vi "Calc Load.vi"(11 "[A/D]":dbl[](array[numeric])) -> (0 "Loads":dbl[](array[numeric]), 1 "Condyle B Load":dbl, 2 "Condyle A Load":dbl, 3 "Total Load":dbl)   [LabVIEW 2015]
uses:
  <vilib>/gmath/NI_Gmath.lvlib
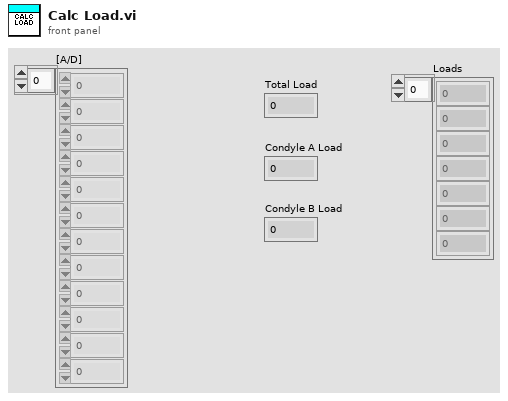
[diagram p1: front panel]
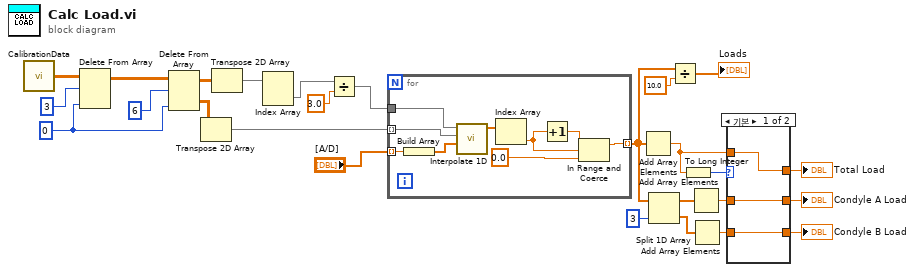
[diagram p0: block diagram]
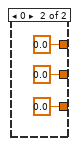
[diagram p2: hidden frame]
diagram:
  w26 = 0 ("index")
  n1 = call "CalibrationData.vi"() -> ("CalData Out"=w4:dbl[][])  [unwired: 1 in]
  n2 = Delete From Array(array=w4, length=3 ("index"), index (col)=w26) -> (array with subset deleted=w24:dbl[][])  [unwired: 1 in, 1 out]
  n3 = Delete From Array(array=w24, length=6, index (col)=w26) -> (deleted portion=w5:dbl[][], array with subset deleted=w22:dbl[][])  [unwired: 1 in]
  n4 = Transpose 2D Array(2D array=w5) -> (transposed array=w18:dbl[][])
  n5 = Transpose 2D Array(2D array=w22) -> (transposed array=w19:dbl[][])
  n6 = Index Array(array=w19) -> (element=w20:dbl[])  [unwired: 2 in]
  n7 = Divide(x=w20, y=3.0 ("Numeric")) -> (x/y=w17:dbl[])
  n8 = for {
    tunnel: w17 -> [w35]
    tunnel: "[A/D]" -> [w34] mode=indexing
    tunnel: [w29] -> w3 mode=indexing
    tunnel: w18 -> [w28] mode=indexing
    n9 = Build Array(w34) -> (w33:dbl[])
    n10 = call <vilib>:"Interpolate 1D.vi"("xi"=w33, "X"=w28, "Y"=w35) -> ("yi"=w32:dbl[])  [unwired: 6 in, 2 out]
    n11 = Index Array(array=w32) -> (element=w31:dbl)  [unwired: 1 in]
    n12 = Increment(x=w31) -> (x+1=w27:dbl)
    n13 = In Range and Coerce(upper limit=w27, x=w31, lower limit=0.0) -> (coerced(x)=w29:dbl)  [unwired: 1 out]
  }
  n14 = Add Array Elements(numeric array=w3) -> (sum=w15:dbl)
  n15 = Split 1D Array(array=w3, index=3) -> (first subarray=w11:dbl[], second subarray=w10:dbl[])
  n16 = Divide(x=w3, y=10.0 ("lower limit")) -> (x/y=→"Loads":dbl[])
  n17 = To Long Integer(number=w15) -> (32bit integer=w16:i32)
  n18 = Add Array Elements(numeric array=w11) -> (sum=w9:dbl)
  n19 = Add Array Elements(numeric array=w10) -> (sum=w8:dbl)
  n20 = case shown="기본" w16 {
    tunnel: w15 -> [w38 _]
    tunnel: [w38 0.0 ("lower limit")] -> w13
    tunnel: w9 -> [w37 _]
    tunnel: w8 -> [w36 _]
    tunnel: [w37 0.0 ("lower limit")] -> w7
    tunnel: [w36 0.0 ("lower limit")] -> w6
    frame Default {
    }
    frame 0 {
    }
  }
  "Total Load" <- w13
  "Condyle A Load" <- w7
  "Condyle B Load" <- w6
